vi "Matlab Param to Matlab String.vi"(8 "error in":errorcluster, 11 "Input Parameter":cluster{"Name":string, "Data":variant}) -> (0 "error out":errorcluster, 3 "Matlab string":string)   [LabVIEW 2010, in "Matlab API.lvlib"]
doc: "This VI converts a Matlab Parameter control item (what is internally used for holding variables to go to or from Matlab) to a string (which is actually sent across the network).\n\nJC 2007-10-25"
uses:
  Matlab API.lvlib
  DBL to Matlab String.vi
  I32 Array to Matlab String.vi
  I32 to Matlab String.vi
  String Array to Matlab String.vi
  String to Matlab String.vi
  Boolean to Matlab String.vi
  Boolean Array to Matlab String.vi
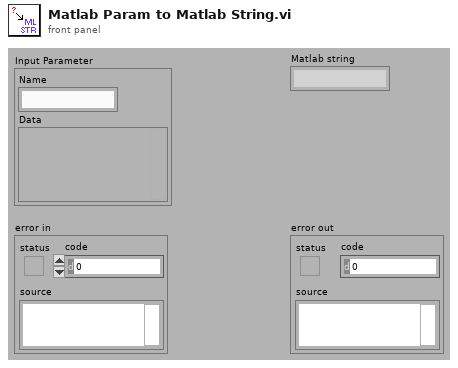
[diagram p1: front panel]
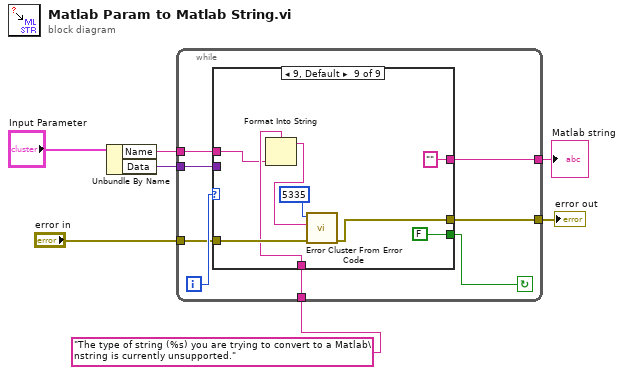
[diagram p0: block diagram]
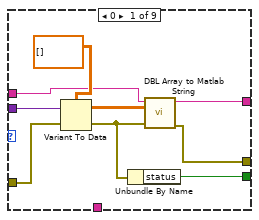
[diagram p2: hidden frame]
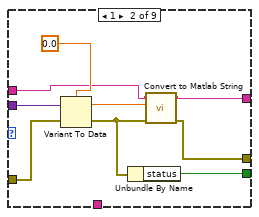
[diagram p3: hidden frame]
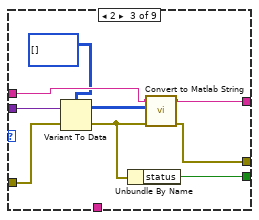
[diagram p4: hidden frame]
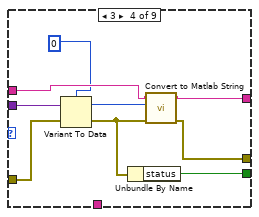
[diagram p5: hidden frame]
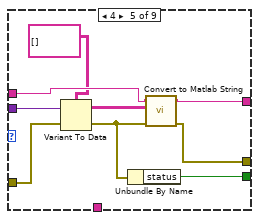
[diagram p6: hidden frame]
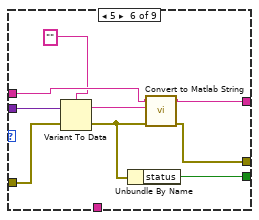
[diagram p7: hidden frame]
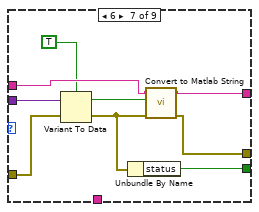
[diagram p8: hidden frame]
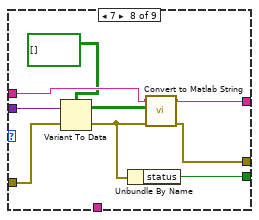
[diagram p9: hidden frame]
diagram:
  n1 = Unbundle By Name("Input Parameter") -> ("Name"=w6:string, "Data"=w5:variant)
  n2 = while {
    tunnel: w6 -> [w14]
    tunnel: w5 -> [w13]
    tunnel: "error in" -> [w12]
    tunnel: [w10] -> w2
    tunnel: [w9] -> w1
    tunnel: "The type of string (%s) you are trying to convert to a Matlab\nstring is currently unsupported." ("error message (\"\")") -> [w8]
    i -> [w15]
    stop <- w11 continue-if-true
    n3 = case shown="9, Default" w15 {
      tunnel: w14 -> [w19 w28 w38 w47 w56 w65 w74 w83 w89]
      tunnel: w13 -> [w24 w33 w42 w51 w60 w69 w78 w87 _]
      tunnel: w12 -> [w23 w32 w41 w50 w59 w68 w77 w86 w95]
      tunnel: [w22 w31 w40 w49 w58 w67 w76 w85 FALSE ("status")] -> w11
      tunnel: [w17 w26 w36 w45 w54 w63 w72 w81 w94] -> w10
      tunnel: [w16 w27 w37 w46 w55 w64 w73 w82 "" ("String")] -> w9
      tunnel: w8 -> [_ _ _ _ _ _ _ _ w90]
      frame 0 {
        n4 = Variant To Data(error in=w23, Variant=w24, type=dbl[][] []) -> (error out=w18:errorcluster, data=w20:dbl[][])
        n5 = Unbundle By Name(w18) -> ("status"=w22:bool)
        n6 = call "DBL Array to Matlab String.vi"("error in (no error)"=w18, "Value"=w20, "Variable name"=w19) -> ("error out"=w17:errorcluster, "String"=w16:string)  [unwired: 7 out]
      }
      frame 1 {
        n7 = Variant To Data(error in=w32, Variant=w33, type=0.0) -> (error out=w25:errorcluster, data=w29:dbl)
        n8 = Unbundle By Name(w25) -> ("status"=w31:bool)
        n9 = call-poly "Convert to Matlab String.vi"("error in (no error)"=w25, "Value"=w29, "Variable name"=w28) -> ("error out"=w26:errorcluster, "String"=w27:string)  [unwired: 7 out]
      }
      frame 2 {
        n10 = Variant To Data(error in=w41, Variant=w42, type=i32[][] []) -> (error out=w35:errorcluster, data=w39:i32[][])
        n11 = Unbundle By Name(w35) -> ("status"=w40:bool)
        n12 = call-poly "Convert to Matlab String.vi"("error in (no error)"=w35, "Value"=w39, "Variable name"=w38) -> ("error out"=w36:errorcluster, "String"=w37:string)  [unwired: 7 out]
      }
      frame 3 {
        n13 = Variant To Data(error in=w50, Variant=w51, type=0) -> (error out=w44:errorcluster, data=w48:i32)
        n14 = Unbundle By Name(w44) -> ("status"=w49:bool)
        n15 = call-poly "Convert to Matlab String.vi"("error in (no error)"=w44, "Value"=w48, "Variable name"=w47) -> ("error out"=w45:errorcluster, "String"=w46:string)  [unwired: 7 out]
      }
      frame 4 {
        n16 = Variant To Data(error in=w59, Variant=w60, type=string[][] []) -> (error out=w53:errorcluster, data=w57:string[][])
        n17 = Unbundle By Name(w53) -> ("status"=w58:bool)
        n18 = call-poly "Convert to Matlab String.vi"("error in (no error)"=w53, "Value"=w57, "Variable name"=w56) -> ("error out"=w54:errorcluster, "String"=w55:string)  [unwired: 7 out]
      }
      frame 5 {
        n19 = Variant To Data(error in=w68, Variant=w69, type="") -> (error out=w62:errorcluster, data=w66:string)
        n20 = Unbundle By Name(w62) -> ("status"=w67:bool)
        n21 = call-poly "Convert to Matlab String.vi"("error in (no error)"=w62, "Value"=w66, "Variable name"=w65) -> ("error out"=w63:errorcluster, "String"=w64:string)  [unwired: 7 out]
      }
      frame 6 {
        n22 = Variant To Data(error in=w77, Variant=w78, type=TRUE) -> (error out=w71:errorcluster, data=w75:bool)
        n23 = Unbundle By Name(w71) -> ("status"=w76:bool)
        n24 = call-poly "Convert to Matlab String.vi"("error in (no error)"=w71, "Data"=w75, "Variable name"=w74) -> ("error out"=w72:errorcluster, "String"=w73:string)  [unwired: 7 out]
      }
      frame 7 {
        n25 = Variant To Data(error in=w86, Variant=w87, type=bool[][] []) -> (error out=w80:errorcluster, data=w84:bool[][])
        n26 = Unbundle By Name(w80) -> ("status"=w85:bool)
        n27 = call-poly "Convert to Matlab String.vi"("error in (no error)"=w80, "Value"=w84, "Variable name"=w83) -> ("error out"=w81:errorcluster, "String"=w82:string)  [unwired: 7 out]
      }
      frame 9, Default {
        n28 = Format Into String(format string=w90, w89) -> (resulting string=w88:string)  [unwired: 2 in, 1 out]
        n29 = call <vilib>:"Error Cluster From Error Code.vi"("error in (no error)"=w95, "error message (\"\")"=w88, "error code (0)"=5335) -> ("error out"=w94:errorcluster)  [unwired: 1 in, 5 out]
      }
    }
  }
  "error out" <- w2
  "Matlab string" <- w1
